vi "Close All Clients.vi"(8 "error in (no error)":errorcluster, 11 "TCP Server in":refnum<class "TCP Server.lvclass">) -> (0 "error out":errorcluster, 2 "Timeout":bool, 3 "TCP Server out":refnum<class "TCP Server.lvclass">)   [LabVIEW 2020, in "Stream-TCP.lvlib" / "TCP Server.lvclass"]
uses:
  TCP Server.lvclass
  TCP Client/TCP Client.lvclass
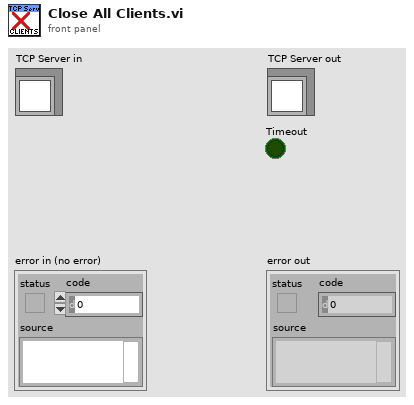
[diagram p1: front panel]
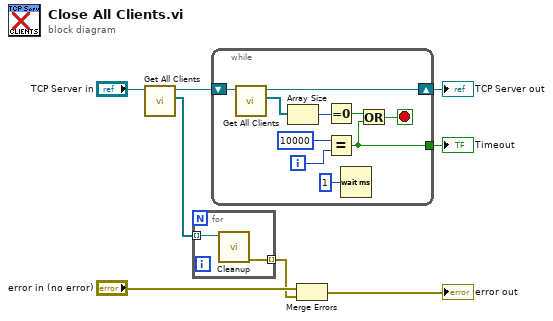
[diagram p0: block diagram]
diagram:
  n1 = call "Get All Clients.vi"("TCP Server in"="TCP Server in") -> ("Clients"=w7:refnum<class "TCP Client.lvclass">[], "TCP Server out"=w3:refnum<class "TCP Server.lvclass">)  [unwired: 8 in, 1 out]
  n2 = for {
    tunnel: w7 -> [w10] mode=indexing
    tunnel: [w9] -> w4 mode=indexing
    n3 = call-dynamic "Cleanup.vi"("TCP Client in"=w10) -> ("error out"=w9:errorcluster)  [unwired: 10 in]
  }
  n4 = while {
    shift-right: [w18] -> w2
    shift-left: w3 -> [w20]
    tunnel: [w12] -> w1
    i -> [w14]
    stop <- w15 stop-if-true
    n5 = call "Get All Clients.vi"("TCP Server in"=w20) -> ("Clients"=w19:refnum<class "TCP Client.lvclass">[], "TCP Server out"=w18:refnum<class "TCP Server.lvclass">)  [unwired: 8 in, 1 out]
    n6 = Array Size(array=w19) -> (size(s)=w17:i32)
    n7 = Equal To 0?(x=w17) -> (x = 0?=w16:bool)
    n8 = Equal?(x=10000, y=w14) -> (x = y?=w12:bool)
    n9 = Wait (ms)(milliseconds to wait=u32 1) -> ()  [unwired: 1 out]
    n10 = Or(x=w16, y=w12) -> (x .or. y?=w15:bool)
  }
  "TCP Server out" <- w2
  "Timeout" <- w1
  n11 = Merge Errors("error in (no error)", w4) -> (→"error out":errorcluster)
